vi "EPOS2N~2.VI"() -> ()   [LabVIEW 2017]
doc: "Example of controlling 1 EPOS2 drive in current mode."
uses:
  <vilib>/addons/Maxon Motor/EPOS2 CANopen/EPOS2 Support Files/Typedefs/EPOS2 Status Word PVM.ctl
  <vilib>/addons/Maxon Motor/EPOS2 CANopen/EPOS2 Support Files/Typedefs/EPOS2 Data Output Current.ctl
  <vilib>/addons/Maxon Motor/EPOS2 CANopen/EPOS2 Support Files/Typedefs/EPOS2 Control Word PVM.ctl
  <vilib>/Platform/TimedLoop/XDataNode/timing_clust.ctl
  <vilib>/Platform/TimedLoop/XDataNode/nitl_modes.ctl
  <vilib>/Platform/TimedLoop/XDataNode/wakeup.ctl
  <vilib>/addons/Maxon Motor/EPOS2 CANopen/EPOS2 Support Files/Polymorphic SubVIs/Write PDO/EPOS2 Current Mode Write.vi
  <vilib>/addons/Maxon Motor/EPOS2 CANopen/EPOS2 Support Files/Polymorphic SubVIs/Read PDO/EPOS2 Current Mode Read.vi
  <vilib>/addons/Maxon Motor/EPOS2 CANopen/CANopen/sbCANopenBaseClass.lvclass
  <vilib>/Platform/TimedLoop/XDataNode/XDataNode.xnode
  <vilib>/Platform/TimedLoop/XDataNode/XDNodeRunTimeDep.lvlib
  <vilib>/addons/Maxon Motor/EPOS2 CANopen/EPOS2 Library.lvlib
panel:
  in  "Switch On":bool=TRUE
  in  "motor":i32
  out "Node ID 3":u8
  out "Data Output":T1
  in  "Current":i32(slide) scale=-1000.0..1000.0
  out "error out":errorcluster
  out "Status":T2
  in  "stop":bool
  # "This Example VI demonstrates how to control the current of an EPOS2 drive using a CANopen interface.\n\nThis VI must be run from a LabVIEW Project. An Example Projects can be found at: \nC:\\Program Files\\National Instruments\\LabVIEW 2015\\examples\\Maxon Motor\\Maxon EPOS2\nor simliar relative path to current LabVIEW version install location for all opperating systems"
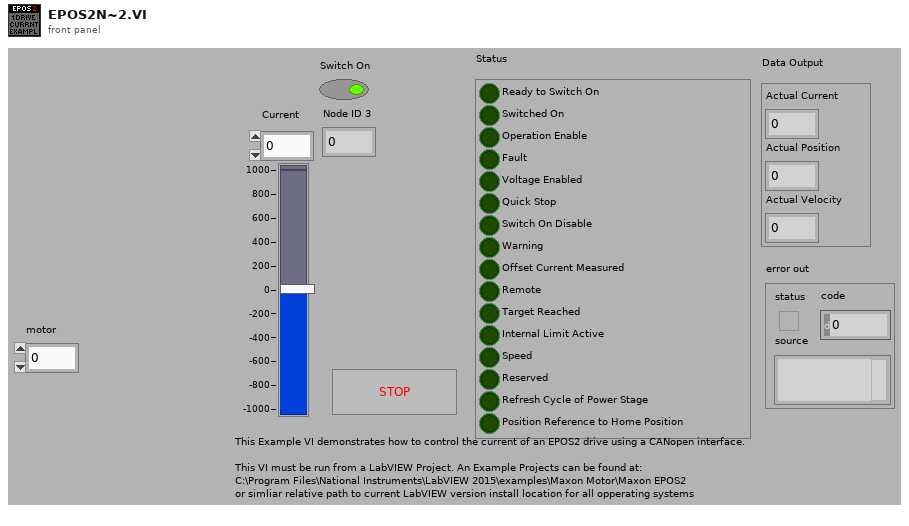
[diagram p1: front panel]
types:
  T1 = typedef "EPOS2 Library.lvlib/EPOS2 Data Output Current.ctl" = cluster{"Actual Current":i16, "Actual Position":i32, "Actual Velocity":i32}
  T2 = typedef "EPOS2 Library.lvlib/EPOS2 Status Word PVM.ctl" = cluster{"Ready to Switch On":bool, "Switched On":bool, "Operation Enable":bool, "Fault":bool, "Voltage Enabled":bool, "Quick Stop":bool, "Switch On Disable":bool, "Warning":bool, "Offset Current Measured":bool, "Remote":bool, "Target Reached":bool, "Internal Limit Active":bool, "Speed":bool, "Reserved":bool, "Refresh Cycle of Power Stage":bool, "Position Reference to Home Position":bool}
  T3 = typedef "EPOS2 Library.lvlib/EPOS2 Control Word PVM.ctl" = cluster{"Switch On":bool, "Enable Voltage":bool, "Quick Stop":bool, "Enable Operation":bool, "Reserved 0":bool, "Reserved 1":bool, "Reserved 2":bool, "Fault Reset":bool, "Halt":bool}
  T4 = typedef "XDNodeRunTimeDep.lvlib/timing_clust.ctl" = cluster{"Expected End [f-1]":u64, "Actual End [f-1]":u64, "Finished Late? [f-1]":bool, "Expected End [i-1]":u64, "Actual End [i-1]":u64, "Finished Late? [i-1]":bool, "Expected Start [i]":u64, "Actual Start [i]":u64, "Expected Start [f]":u64, "Actual Start [f]":u64, "Source Name":string, "Structure Name":string, "Period":i64, "Deadline":i64, "Offset":i64, "Start":i64, "Priority":i32, "Timeout":i32, "Mode":T5, "Wakeup Reason":T6, "Error":errorcluster, "Source Type":string, "Secondary Source Type":string, "Global End Time":u64, "Global Start Time":u64, "Frame Duration":u64, "Iteration Duration":u64, "Assigned CPU":i32, "I/O Scan Engine Mode":u32}
  T5 = typedef "XDNodeRunTimeDep.lvlib/nitl_modes.ctl" = enum32{"No Change", "Process missed periods, maintain original phase", "Discard missed periods, maintain original phase", "Process missed periods, ignore original phase", "Discard missed periods, ignore original phase"}
  T6 = typedef "XDNodeRunTimeDep.lvlib/wakeup.ctl" = enum32{"Normal", "Aborted", "Asynchronous wakeup", "Timing source error", "Timed loop error", "Timeout"}
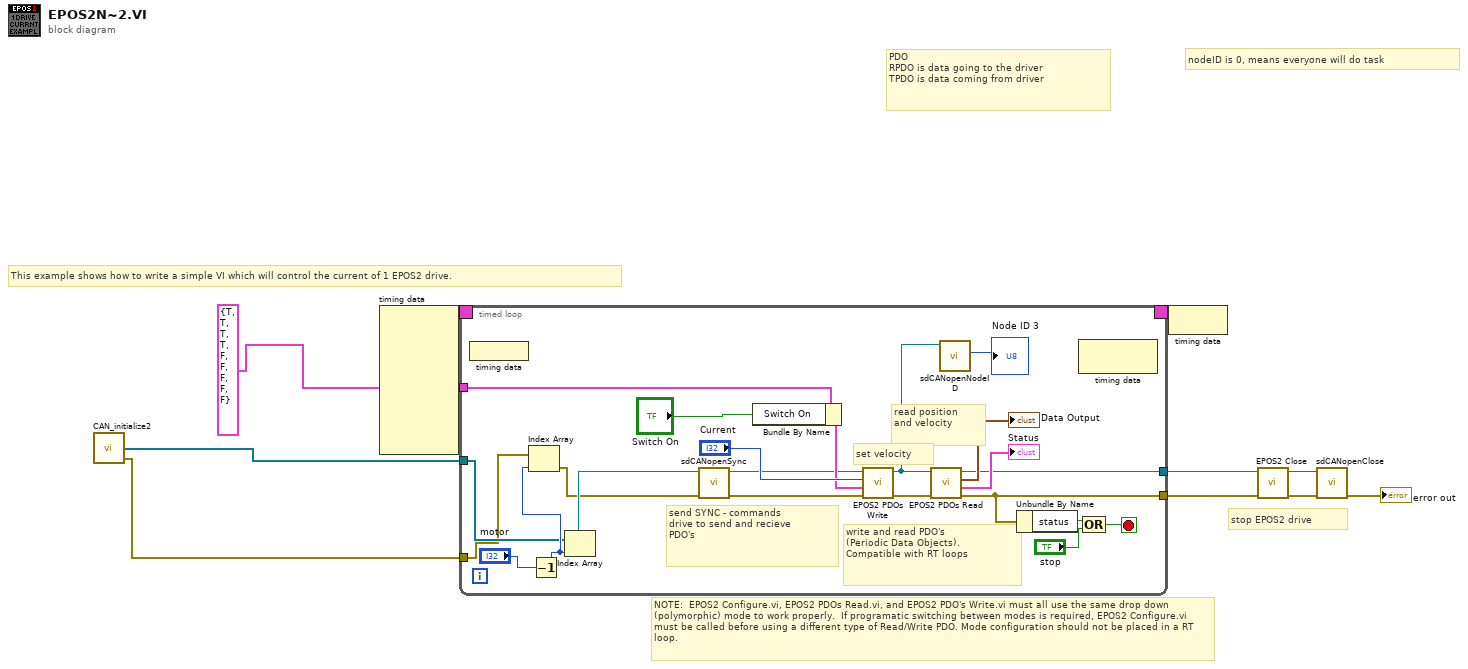
[diagram p0: block diagram]
diagram:
  # "nodeID is 0, means everyone will do task"
  # "PDO\nRPDO is data going to the driver\nTPDO is data coming from driver"
  # "This example shows how to write a simple VI which will control the current of 1 EPOS2 drive."
  # "stop EPOS2 drive"
  # "NOTE:  EPOS2 Configure.vi, EPOS2 PDOs Read.vi, and EPOS2 PDO's Write.vi must all use the same drop down (polymorphic) mode to work properly.  If programatic switching between modes is required, EPOS2 Configure.vi must be called before using a different type of Read/Write PDO. Mode configuration should not be placed in a RT loop."
  n1 = call "CAN_initialize2.vi"() -> ("Array 2"=w2:errorcluster[], "Array"=w3:refnum<class "sbCANopenBaseClass.lvclass">[])  [unwired: 3 in, 1 out]
  n2 = node-c288() -> (w10:T4)  [unwired: 6 in, 2 out]
  n3 = timed-loop {
    timing: w10 -> [_]
    timing-out: [_] -> w9
    tunnel: T3 {"Switch On"=TRUE, "Enable Voltage"=TRUE, "Quick Stop"=TRUE, "Enable Operation"=TRUE, "Reserved 0"=FALSE, "Reserved 1"=FALSE, "Reserved 2"=FALSE, "Fault Reset"=FALSE, "Halt"=FALSE} ("Control Word") -> [w26]
    tunnel: [w18] -> w5
    tunnel: [w13] -> w4
    tunnel: w3 -> [w12]
    tunnel: w2 -> [w11]
    stop <- w23 stop-if-true
    # "read position\nand velocity"
    # "set velocity"
    # "write and read PDO's\n(Periodic Data Objects).\nCompatible with RT loops"
    # "send SYNC - commands\ndrive to send and recieve\nPDO's"
    n4 = node-c288() -> ()  [unwired: 1 out]
    n5 = Decrement(x="motor") -> (x-1=w15:i32)
    n6 = Index Array(array=w11, index=w15) -> (element=w14:errorcluster)
    n7 = Index Array(array=w12, index=w15) -> (element=w19:refnum<class "sbCANopenBaseClass.lvclass">)
    n8 = call-dynamic "sdCANopenSync.vi"("error in (no error)"=w14, "sbCANopenBaseClass in"=w19) -> ("error out"=w30:errorcluster, "sbCANopenBaseClass out"=w22:refnum<class "sbCANopenBaseClass.lvclass">)  [unwired: 8 in]
    n9 = Bundle By Name(cluster=w26, "Switch On"="Switch On") -> (w25:T3)
    n10 = call-poly <vilib>:"EPOS2 PDOs Write.vi"("error in"=w30, "Control Word"=w25, "Current"="Current", "CANopen Session In"=w22) -> ("error out"=w29:errorcluster, "CANopen Session Out"=w20:refnum<class "sbCANopenBaseClass.lvclass">)  [unwired: 6 in]
    n11 = call-poly <vilib>:"EPOS2 PDOs Read.vi"("error in"=w29, "CANopen Session In"=w20) -> ("error out"=w13:errorcluster, "Statusword"=→"Status":T2, "Data Output"=→"Data Output":T1, "CANopen Session Out"=w18:refnum<class "sbCANopenBaseClass.lvclass">)  [unwired: 6 in]
    n12 = call-dynamic "sdCANopenNodeID.vi"("sbCANopenBaseClass in"=w20) -> ("Node ID"=→"Node ID 3":u8)  [unwired: 9 in, 1 out]
    n13 = Unbundle By Name(w13) -> ("status"=w31:bool)
    n14 = node-c288() -> ()  [unwired: 2 out]
    n15 = Compound Arithmetic op=OR(w31, "stop") -> (w23:bool)
  }
  n16 = node-c288(w9) -> ()
  n17 = call <vilib>:"EPOS2 Close.vi"("error in"=w4, "CANopen Session In"=w5) -> ("error out"=w7:errorcluster, "CANopen Session Out"=w8:refnum<class "sbCANopenBaseClass.lvclass">)  [unwired: 2 in, 6 out]
  n18 = call-dynamic "sdCANopenClose.vi"("error in (no error)"=w7, "sbCANopenBaseClass in"=w8) -> ("error out"=→"error out":errorcluster)  [unwired: 8 in, 1 out]
